vi "SavePyFile.vi"(7 "Name":string="Main.py", 8 "error in":errorcluster, 9 "Console In":string, 10 "Python Code":string, 11 "VISA in":refnum<visa-resource-name>) -> (0 "error out":errorcluster, 1 "Reply":string, 3 "VISA out":refnum<visa-resource-name>)   [LabVIEW 2016]
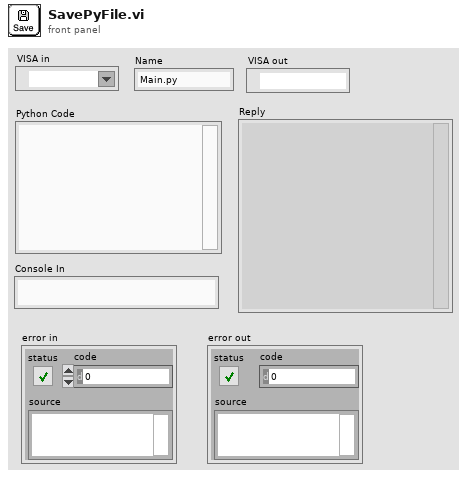
[diagram p1: front panel]
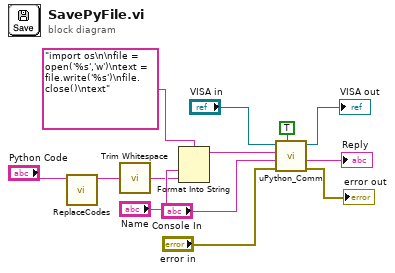
[diagram p0: block diagram]
diagram:
  n1 = call "ReplaceCodes.vi"("String in"="Python Code") -> ("Conv String out"=w1:string)  [unwired: 9 in, 1 out]
  n2 = call <vilib>:"Trim Whitespace.vi"("string"=w1) -> ("trimmed string"=w11:string)  [unwired: 1 in]
  n3 = Format Into String(format string="import os\n\nfile = open('%s','w')\ntext = file.write('%s')\nfile.close()\ntext" ("write buffer"), "Name", w11) -> (resulting string=w12:string)  [unwired: 2 in, 1 out]
  n4 = call "uPython_Comm.vi"("Wait for Reply?"=TRUE, "error in (no error)"="error in", "Console In"="Console In", "Script"=w12, "VISA Refnum in"="VISA in") -> ("error out"=→"error out":errorcluster, "Console Out"=→"Reply":string, "VISA out"=→"VISA out":refnum<visa-resource-name>)  [unwired: 2 in, 2 out]
